vi "1 Helper - Wind calculator.vi"(8 "Robot Velocity":T2 {"East" format="%#_5g"}, 9 "Heading":T1 format="%05.1f", 10 "Absolute Wind Direction":T1=45.0 format="%05.1f", 11 "Absolute Wind Speed":dbl=1.0) -> (0 "Apparent Wind Direction":T1 format="%05.1f", 1 "Apparent Wind Speed":T3, 2 "Absolute Wind Direction":T1 format="%05.1f", 3 "Absolute Wind Speed":dbl)   [LabVIEW 2011]
uses:
  2-Think/2 Typedefs/heading.ctl
  2-Think/2 Typedefs/Velocity.ctl
  2-Think/2 Typedefs/apparent wind speed.ctl
  2-Think/2 Globals/2 Global.vi
panel:
  out "Apparent Wind\nin global ref frame":T2 {"East" format="%#_5g"}
  out "Absolute Wind":T2 {"East" format="%#_5g"}
  in  "Add Randomness\nTo Wind Measurement":bool
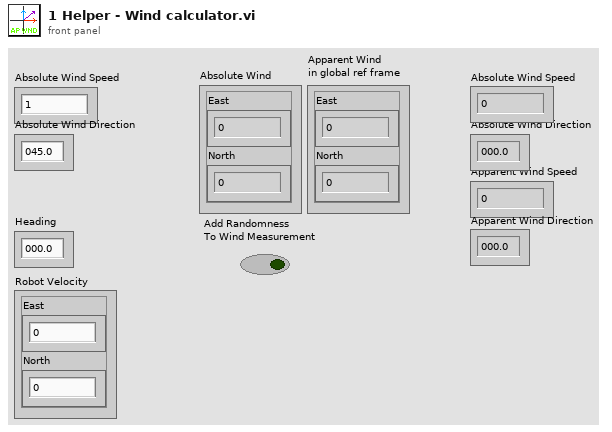
[diagram p1: front panel]
types:
  T1 = typedef "heading.ctl" = dbl
  T2 = typedef "Velocity.ctl" = cluster{"East":dbl, "North":dbl}
  T3 = typedef "apparent wind speed.ctl" = dbl
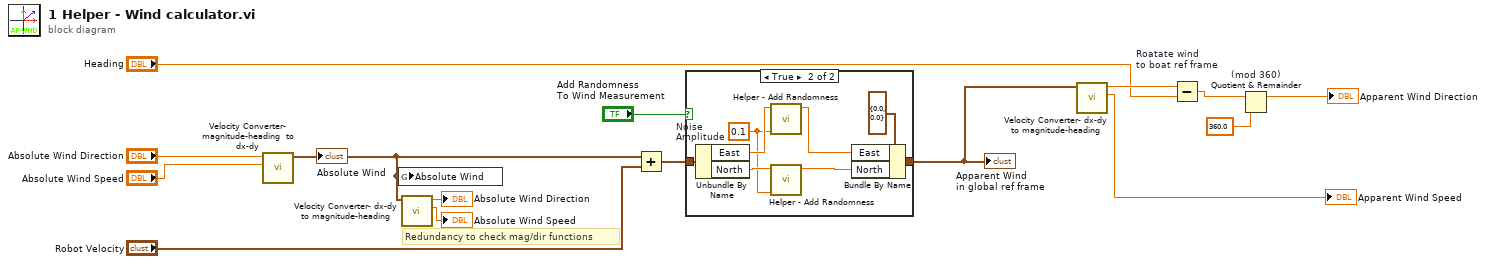
[diagram p0: block diagram]
diagram:
  # "Redundancy to check mag/dir functions"
  n1 = call "Velocity Converter- magnitude-heading  to dx-dy.vi"("Magnitude"="Absolute Wind Speed", "Heading"="Absolute Wind Direction") -> ("Vector Out"=w5:T2)  [unwired: 9 in]
  "Absolute Wind" <- w5
  n2 = global write "2 Global.vi" "Absolute Wind"(w5) -> ()
  n3 = call "Velocity Converter- dx-dy to magnitude-heading.vi"("Vector In"=w5) -> ("Magnitude Out"=→"Absolute Wind Speed":dbl, "Heading Out"=→"Absolute Wind Direction":T1)  [unwired: 9 in]
  n4 = Add(x=w5, y="Robot Velocity") -> (x+y=w9:T2)
  n5 = case shown="True" "Add Randomness\nTo Wind Measurement" {
    tunnel: [w16 w24] -> w11
    tunnel: w9 -> [w16 w23]
    frame False {
    }
    frame True {
      w18 = 0.1  # Noise Amplitude
      n6 = Unbundle By Name(w23) -> ("East"=w22:dbl, "North"=w21:dbl)
      n7 = call "Helper - Add Randomness.vi"("Amplitude\n(default 1)"=w18, "Numeric in"=w22) -> ("Numeric out"=w19:dbl)  [unwired: 9 in]
      n8 = call "Helper - Add Randomness.vi"("Amplitude\n(default 1)"=w18, "Numeric in"=w21) -> ("Numeric out"=w20:dbl)  [unwired: 9 in]
      n9 = Bundle By Name(cluster=T2 {"East"=0.0, "North"=0.0} ("Apparent Wind 2"), "East"=w19, "North"=w20) -> (w24:T2)
    }
  }
  "Apparent Wind\nin global ref frame" <- w11
  n10 = call "Velocity Converter- dx-dy to magnitude-heading.vi"("Vector In"=w11) -> ("Magnitude Out"=→"Apparent Wind Speed":dbl, "Heading Out"=w6:T1)  [unwired: 9 in]
  n11 = Subtract "Roatate wind\nto boat ref frame"(x=w6, y="Heading") -> (x-y=w10:T1)
  n12 = Quotient & Remainder "(mod 360)"(x=w10, y=T1 360.0) -> (x-y*floor(x/y)=→"Apparent Wind Direction":T1)  [unwired: 1 out]
